vi "Read Captains.vi"(8 "error in (no error)":errorcluster, 11 "Captains":path) -> (0 "error out":errorcluster, 3 "Captains":string[](array[string]))   [LabVIEW 2021, in "Ship.lvclass"]
uses:
  Ship.lvclass
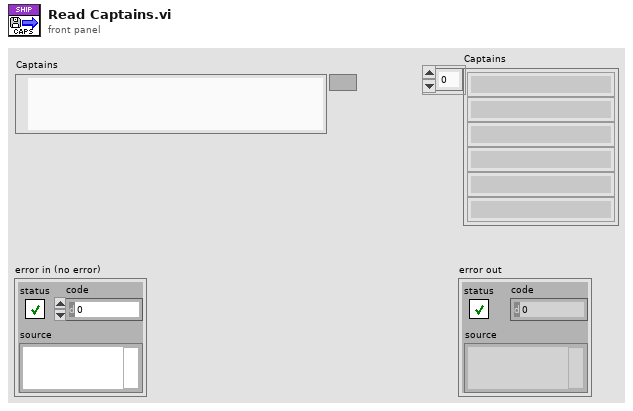
[diagram p1: front panel]
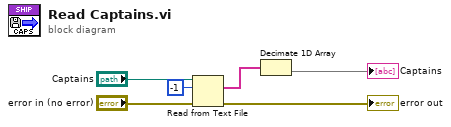
[diagram p0: block diagram]
diagram:
  n1 = Read from Text File(file (use dialog)="Captains", count=-1, error in="error in (no error)") -> (text=w3:string[], error out=→"error out":errorcluster)  [unwired: 1 in, 2 out]
  n2 = Decimate 1D Array(w3) -> (→"Captains":string[])  [unwired: 1 out]
